vi "XW_Tutu_Chevray.vi"() -> (5 "Plug in titles":string[](array[string]), 7 "Plug in values":string[](array[string]))   [LabVIEW 2021]
uses:
  Controls/Inst_type.ctl
  Controls/In_Range.ctl
  Globals/Meas_global.vi
  <vilib>/Utility/file.llb/Read From Spreadsheet File (string).vi
panel:
  out "Calib Index":i32
  out "Third":dbl format="%#.3f"
  out "Filename":string
  out "Third Component":path
  out "U index":i32
  out "Log Row":i32
  out "2nd Comp":string
  out "1st Comp":string
  out "Iterations":i32
  out "Results table":string[][](table)
  out "Psi 2":dbl=-999.0 format="%.2f"
  out "Psi 1":dbl=-999.0 format="%.2f"
  out "UW":bool
  in  "constants":T1={"u'/U"=0.5, "v'/U"=0.4, "w'/U"=0.4, "rho"=0.5, "alpha1"=0.0, "alpha2"=0.0} {"alpha2" format="%.2f"; "alpha1" format="%.2f"; "rho" format="%.2f"; "w'/U" format="%.2f"; "v'/U" format="%.2f"; "u'/U" format="%.2f"}
  in  "u*, v* limits":T2={"u* low"=0.4, "u* high"=1.8, "v* low"=-0.6, "v* high"=0.8} {"v* high" format="%.2f"; "v* low" format="%.2f"; "u* high" format="%.2f"; "u* low" format="%.2f"}
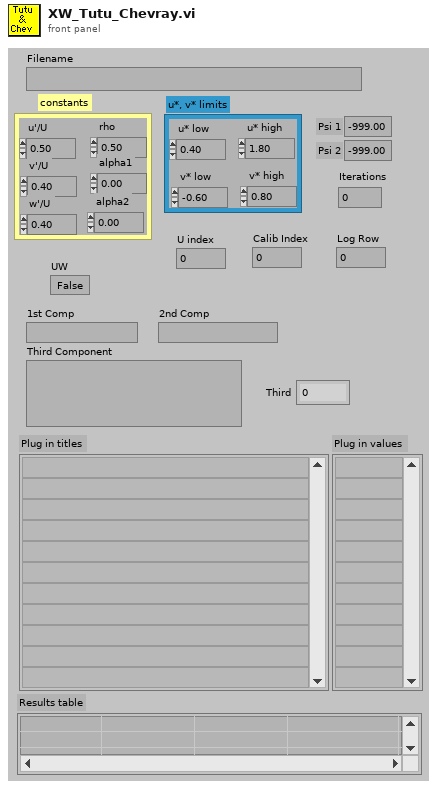
[diagram p1: front panel]
types:
  T1 = cluster{"u'/U":dbl, "v'/U":dbl, "w'/U":dbl, "rho":dbl, "alpha1":dbl, "alpha2":dbl}
  T2 = cluster{"u* low":dbl, "u* high":dbl, "v* low":dbl, "v* high":dbl}
  T3 = typedef "Analysis_info_cluster.ctl" = cluster{"Colour":u32, "Inst type":T4, "Inst name":string, "Symbol":string, "Code name":string, "Extra Info":string, "Inst Array":T5, "Extra Titles":string[], "Extra Values":string[], "U":dbl, "u^2":dbl, "u^3":dbl, "u^4":dbl, "Skew_u":dbl, "Kurt_u":dbl, "Sd Error in Mean":dbl, "% u'/U":dbl, "X":dbl, "Y":dbl, "Z":dbl, "Timescale integral Estimate":dbl, "Sd Error in Variance":dbl, "Calib File":path, "Calib Constants":dbl[], "Output Position":bool, "Stats":enum16{"None", "Basic", "Full"}, "Av Sampling Rate":dbl, "Av No of Samples":dbl, "Total Meas Time (s)":dbl, "ADAM Ch Name":string, "Max value":dbl, "Min value":dbl, "Req Sample Rate Hz":dbl, "Sync Delay Time (s)":dbl, "Ch No":i16, "Device":string, "Use Latest Calib":bool, "Port":string, "Metadata Ch Names":string[], "Metadata Ch Values":string[], "Label":string}
  T4 = typedef "Inst_type.ctl" = enum16{"Raw voltage", "Raw with zero offsetting", "Propeller anemometer", "Pressure Transducer", "Pitot-static tube", "Hot wire", "Cross wire 1", "Cross wire 2", "Generic Linear", "Generic Polynomial", "Generic BackPoly", "Fast FID", "Thermocouple", "Cold wire", "Pulsed Wire", "LDA Vel", "LDA Tran time", "LDA Arr time", "Microphone"}
  T5 = typedef "Instrument_Array.ctl" = enum16{"PWA", "LDA", "Analogue"}
  T6 = typedef "In_Range.ctl" = enum16{"%", "±", "% & ±"}
  T7 = enum16{"Save no data", "Save data in new files", "Save data in existing files"}
  T8 = typedef "Time_Trace_Cluster.ctl" = cluster{"Weighting":dbl[], "Voltage":dbl[], "Eng Values":dbl[]}
  T9 = typedef "Cross_Moments_Shift_Cluster.ctl" = cluster{"Stats":dbl[], "Resampled No of Samples":i32, "Resampled delta T":dbl, "Cross Correlation":dbl[]}
  T10 = typedef "Shift_Cluster.ctl" = cluster{"Stats":dbl[], "Spectra_Auto":dbl[], "Histogram":dbl[], "Hist Max":dbl, "Hist Min":dbl, "No of Samples":i32, "No in plume":i32, "Weight sum":dbl, "No Of Hist bins":i32, "TimeTrace Max":dbl, "Time Trace Min":dbl, "Trace St Deviation":dbl}
  T11 = typedef "Correlation_cluster1.ctl" = cluster{"U inst":string, "uw":dbl, "u^2w":dbl, "uw^2":dbl, "uw/u'w'":dbl, "W inst":string, "uw^3":dbl, "u^3w":dbl, "u^2w^2":dbl, "Index U":i32, "Index W":i32, "Error info":string[], "Paired Sampling Rate (Hz)":dbl, "u^2 Paired":dbl, "w^2 Paired":dbl, "Time Window (ms)":dbl}
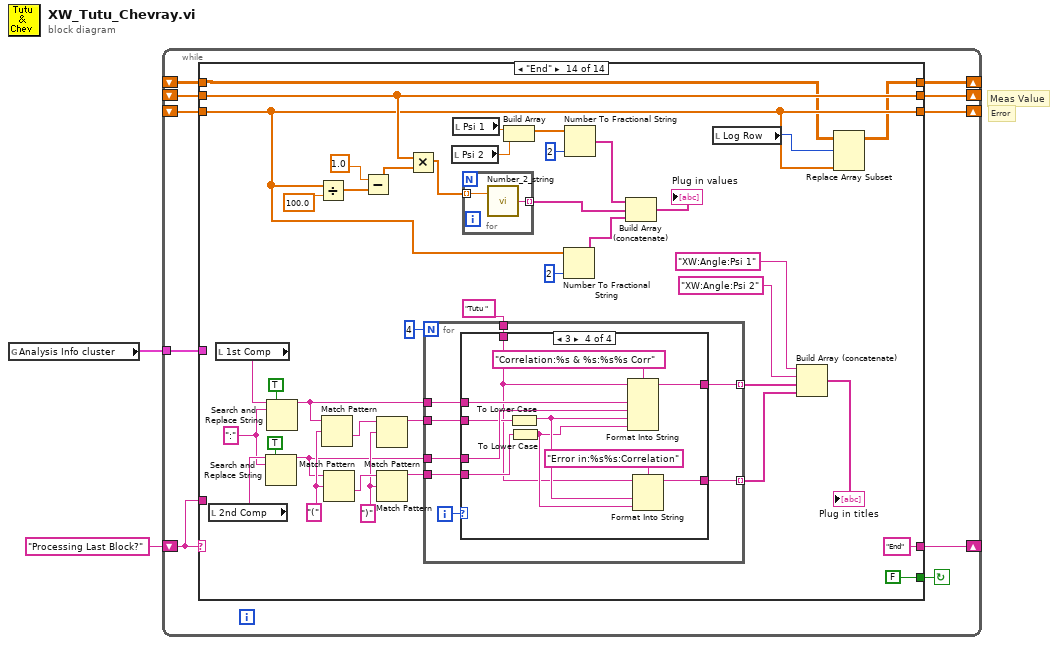
[diagram p0: block diagram]
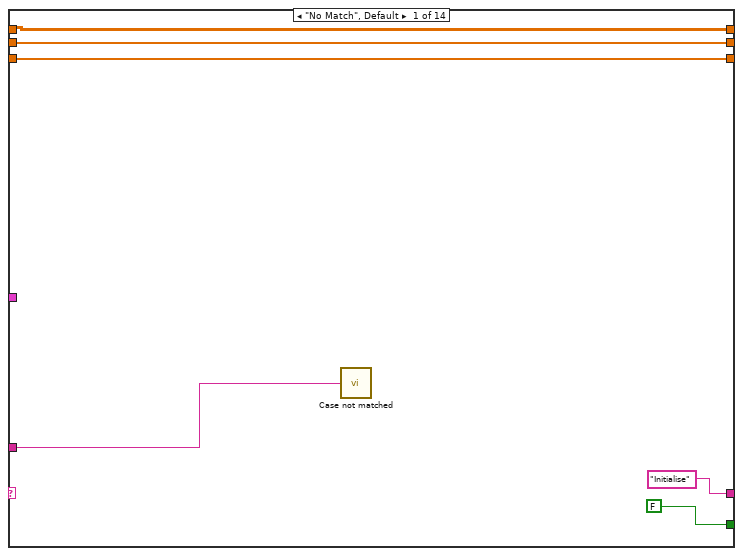
[diagram p2: hidden frame]
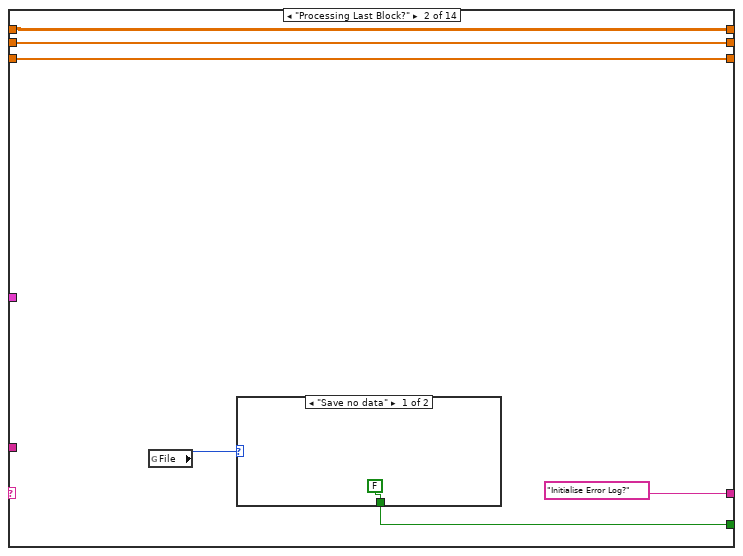
[diagram p3: hidden frame]
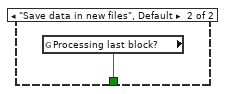
[diagram p4: hidden frame]
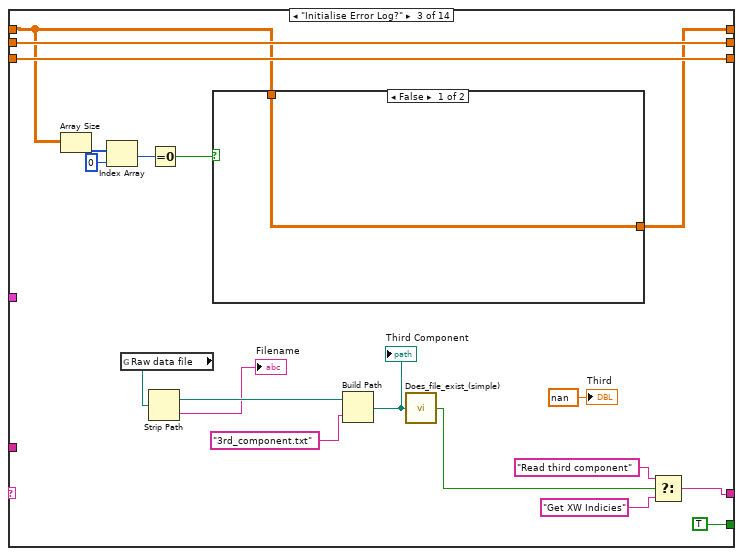
[diagram p5: hidden frame]
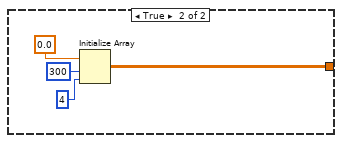
[diagram p6: hidden frame]
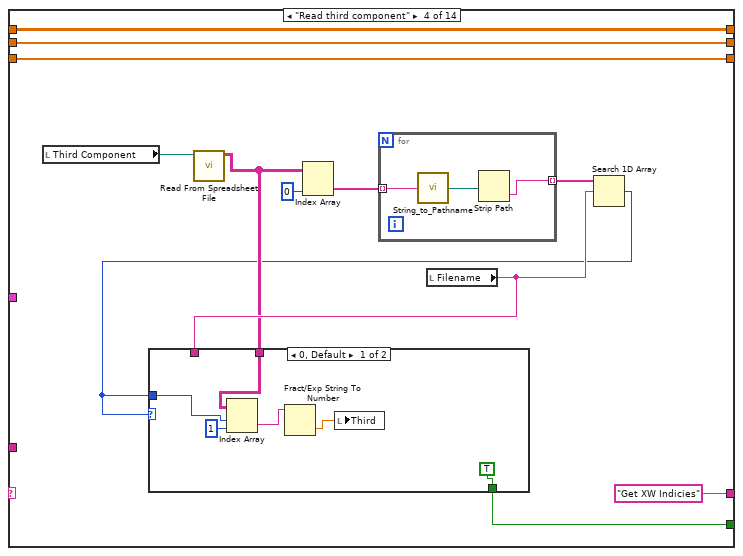
[diagram p7: hidden frame]
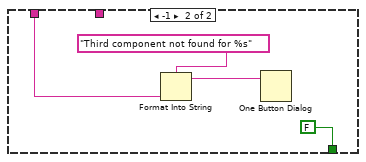
[diagram p8: hidden frame]
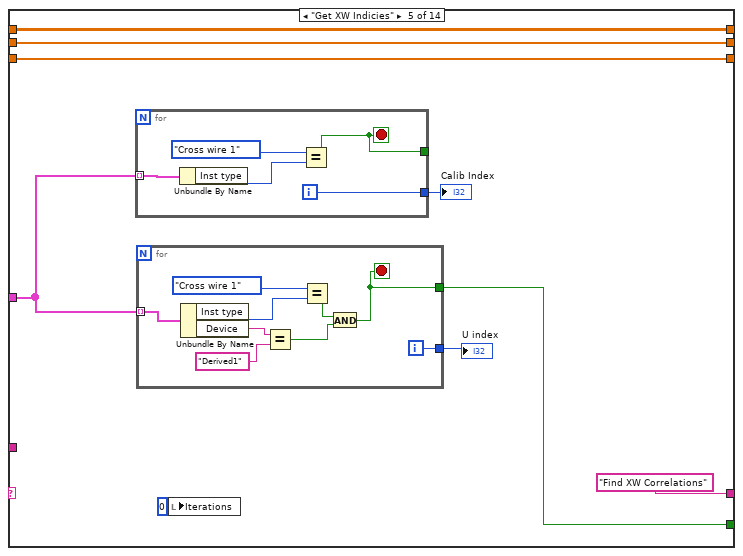
[diagram p9: hidden frame]
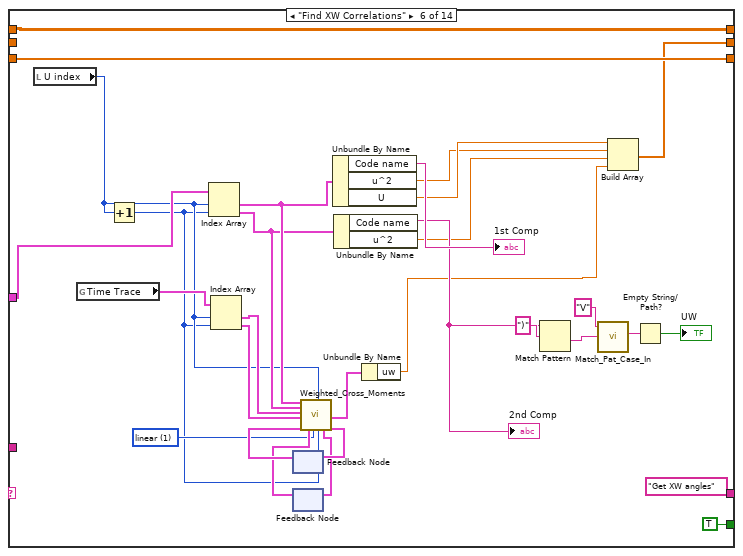
[diagram p10: hidden frame]
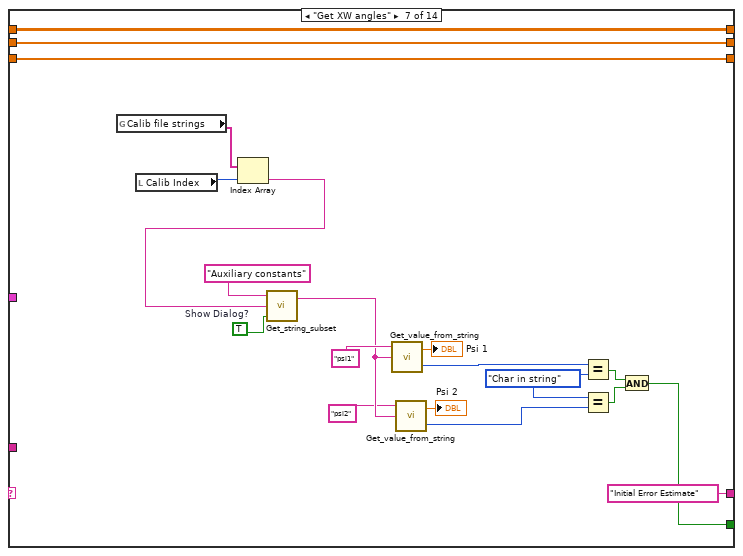
[diagram p11: hidden frame]
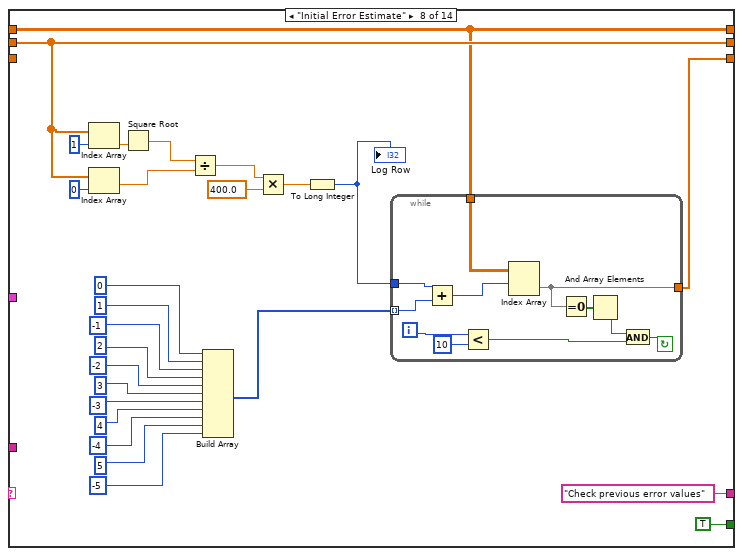
[diagram p12: hidden frame]
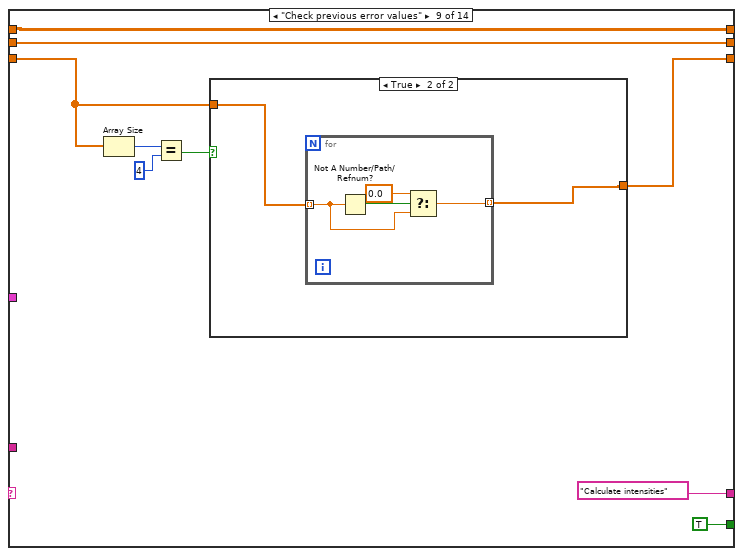
[diagram p13: hidden frame]
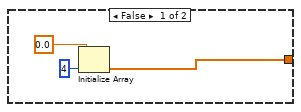
[diagram p14: hidden frame]
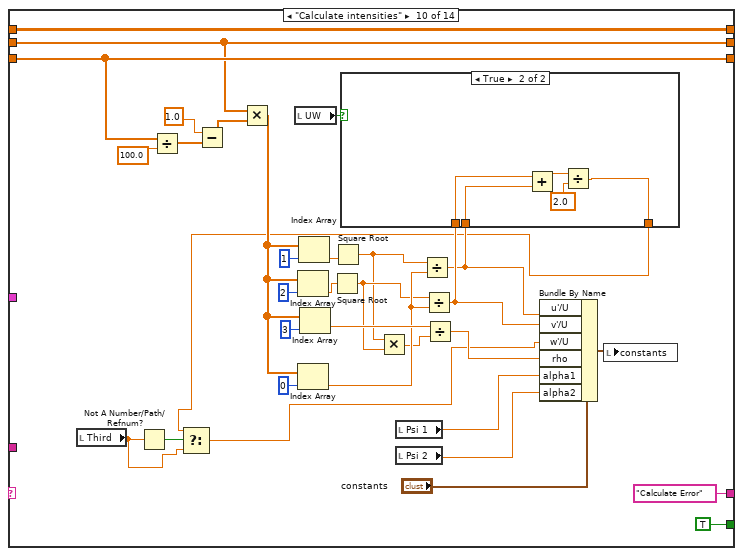
[diagram p15: hidden frame]
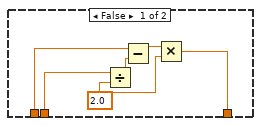
[diagram p16: hidden frame]
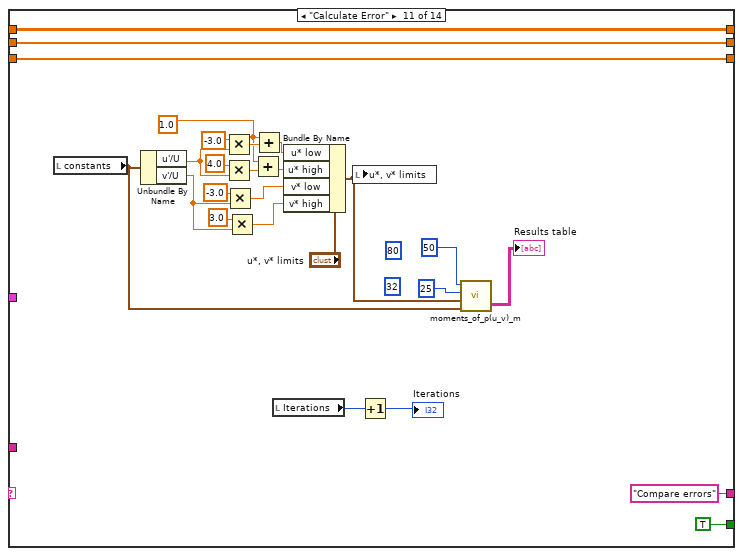
[diagram p17: hidden frame]
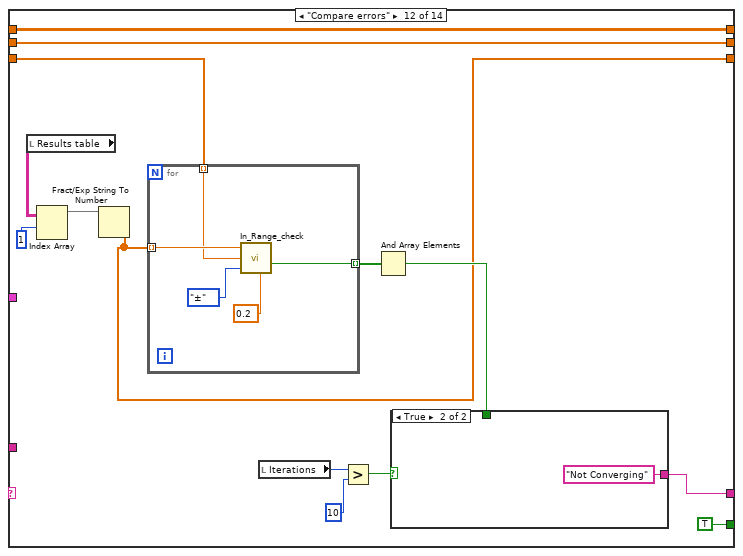
[diagram p18: hidden frame]
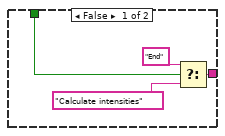
[diagram p19: hidden frame]
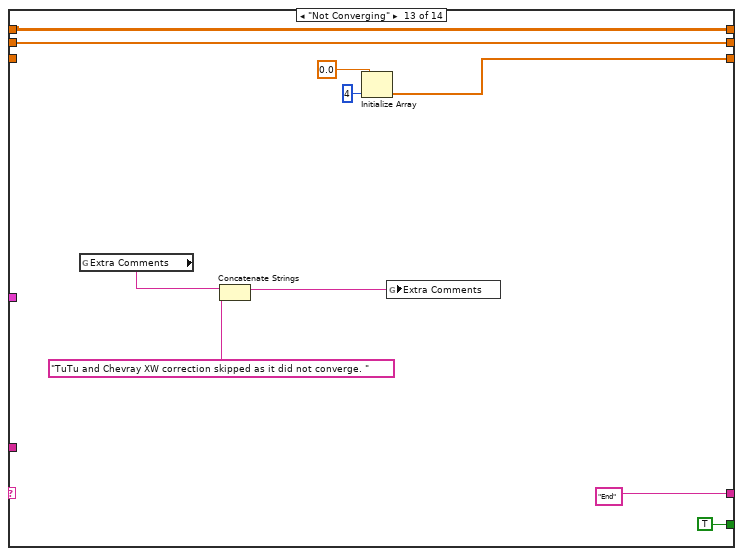
[diagram p20: hidden frame]
diagram:
  # "Error"
  # "Meas Value"
  n1 = global read "Meas_global.vi" "Analysis Info cluster"() -> (w1:T3[])
  n2 = while {
    tunnel: w1 -> [w6]
    shift-left: _ -> [w5]
    shift-right: [w7] -> _
    shift-left: _ -> [w8]
    shift-right: [w9] -> _
    shift-left: "Processing Last Block?" -> [w10]
    shift-right: [w11] -> _
    shift-right: [w3] -> _
    shift-left: _ -> [w4]
    stop <- w12 continue-if-true
    n3 = case shown="\"End\"" w10 {
      tunnel: [FALSE w23 TRUE ("Processing last block?") w53 w77 TRUE ("Processing last block?") w131 TRUE ("Processing last block?") TRUE ("Processing last block?") TRUE ("Processing last block?") TRUE ("Processing last block?") TRUE ("Processing last block?") TRUE ("Processing last block?") FALSE ("Processing last block?")] -> w12
      tunnel: ["Initialise" "Initialise Error Log?" w29 "Get XW Indicies" "Find XW Correlations" "Get XW angles" "Initial Error Estimate" "Check previous error values" ("f") "Calculate intensities" "Calculate Error" "Compare errors" w282 "End" "End"] -> w11
      tunnel: w10 -> [w13 _ _ _ _ _ _ _ _ _ _ _ _ _]
      tunnel: [w16 w22 w45 w61 w83 w119 w139 w167 w194 w228 w273 w287 w307 w342] -> w9
      tunnel: w8 -> [w16 w22 w45 w61 w83 _ w139 w167 w194 w228 w273 w287 w307 w342]
      tunnel: [w15 w20 w44 w60 w82 w127 w138 w161 w190 w233 w253 w278 w303 w321] -> w7
      tunnel: w6 -> [_ _ _ _ w79 w114 _ _ _ _ _ _ _ _]
      tunnel: w5 -> [w15 w20 w44 w60 w82 w127 w138 _ w189 w233 w253 w285 _ w321]
      tunnel: [w14 w19 w38 w62 w81 w115 w130 w163 w187 w208 w248 w274 w298 w320] -> w3
      tunnel: w4 -> [w14 w19 w37 w62 w81 w115 w130 w163 w187 w208 w248 w274 w298 w319]
      frame "No Match", Default {
        n4 = call "Case not matched.vi"("Case Name not Matched"=w13) -> ()
      }
      frame "Processing Last Block?" {
        n5 = global read "Meas_global.vi" "File"() -> (w21:T7)
        n6 = case shown="\"Save no data\"" w21 {
          tunnel: [FALSE ("Processing last block?") w26] -> w23
          frame "Save no data" {
          }
          frame "Save data in new files", Default {
            n7 = global read "Meas_global.vi" "Processing last block?"() -> (w26:bool)
          }
        }
      }
      frame "Initialise Error Log?" {
        n8 = Array Size(array=w37) -> (size(s)=w42:i32[])
        n9 = Index Array(array=w42, index=0) -> (element=w40:i32)
        n10 = global read "Meas_global.vi" "Raw data file"() -> (w36:path)
        n11 = Strip Path(path=w36) -> (stripped path=w35:path, name=→"Filename":string)
        n12 = Equal To 0?(x=w40) -> (x = 0?=w39:bool)
        n13 = case shown="False" w39 {
          tunnel: [w46 w47] -> w38
          tunnel: w37 -> [w46 _]
          frame False {
          }
          frame True {
            n14 = Initialize Array(0.0, 300 ("dimension size"), 4 ("dimension size")) -> (w47:dbl[][])
          }
        }
        n15 = Build Path(base path=w35, name or relative path="3rd_component.txt") -> (appended path=w33:path)
        "Third Component" <- w33
        n16 = call "Does_file_exist_(simple).vi"("Pathname"=w33) -> ("exists?"=w30:bool)
        n17 = Select(t="Read third component", s=w30, f="Get XW Indicies") -> (s? t:f=w29:string)
        "Third" <- nan ("Third")
      }
      frame "Read third component" {
        n18 = local read "Third Component"() -> (w58:path)
        n19 = call-poly <vilib>:"Read From Spreadsheet File.vi"("file path (dialog if empty)"=w58) -> ("all rows"=w52:string[][])  [unwired: 3 in, 7 out]
        n20 = Index Array(array=w52, index (col)=0 ("disabled index (col)")) -> (element=w56:string[])  [unwired: 1 in]
        n21 = for {
          tunnel: w56 -> [w75] mode=indexing
          tunnel: [w73] -> w55 mode=indexing
          n22 = call "String_to_Pathname.vi"("Input String"=w75) -> ("path"=w74:path)
          n23 = Strip Path(path=w74) -> (name=w73:string)  [unwired: 1 out]
        }
        n24 = local read "Filename"() -> (w54:string)
        n25 = Search 1D Array(1D array=w55, element=w54) -> (index of element=w51:i32)  [unwired: 1 out]
        n26 = case shown="0, Default" w51 {
          tunnel: w54 -> [_ w72]
          tunnel: [TRUE ("Processing last block?") FALSE ("Processing last block?")] -> w53
          tunnel: w52 -> [w66 _]
          tunnel: w51 -> [w65 _]
          frame 0, Default {
            n27 = Index Array(array=w66, index (row)=w65, index (col)=1 ("disabled index (col)")) -> (element=w64:string)
            n28 = Fract/Exp String To Number(string=w64) -> (number=w63:dbl)  [unwired: 4 out]
            n29 = local write "Third"(w63) -> ()
          }
          frame -1 {
            n30 = Format Into String(format string="Third component not found for %s" ("message"), w72) -> (resulting string=w70:string)  [unwired: 2 in, 1 out]
            n31 = One Button Dialog(message=w70) -> ()  [unwired: 2 out]
          }
        }
      }
      frame "Get XW Indicies" {
        n32 = for {
          tunnel: [w95] -> _
          tunnel: w79 -> [w97] mode=indexing
          tunnel: [w94] -> w76
          i -> [w94]
          stop <- w95 stop-if-true
          n33 = Unbundle By Name(w97) -> ("Inst type"=w98:T4)
          n34 = Equal?(x=Inst_type."Cross wire 1" ("Inst type"), y=w98) -> (x = y?=w95:bool)
        }
        "Calib Index" <- w76
        n35 = for {
          tunnel: [w86] -> w77
          tunnel: w79 -> [w92] mode=indexing
          tunnel: [w85] -> w78
          i -> [w85]
          stop <- w86 stop-if-true
          n36 = Unbundle By Name(w92) -> ("Inst type"=w93:T4, "Device"=w90:string)
          n37 = Equal?(x=w90, y="Derived1") -> (x = y?=w87:bool)
          n38 = Equal?(x=Inst_type."Cross wire 1" ("Inst type"), y=w93) -> (x = y?=w88:bool)
          n39 = And(x=w88, y=w87) -> (x .and. y?=w86:bool)
        }
        "U index" <- w78
        n40 = local write "Iterations"(0 ("Iterations")) -> ()
      }
      frame "Find XW Correlations" {
        w101 = 1 items=["nearest", "linear", "spline", "cubic Hermite", "Lagrange"] ("interp. method")
        n41 = local read "U index"() -> (w100:i32)
        n42 = global read "Meas_global.vi" "Time Trace"() -> (w113:T8[])
        n43 = Increment(x=w100) -> (x+1=w99:i32)
        n44 = Index Array(array=w114, index #1=w100, index #2=w99) -> (element #1=w112:T3, element #2=w111:T3)
        n45 = Index Array(array=w113, index #1=w100, index #2=w99) -> (element #1=w110:T8, element #2=w109:T8)
        n46 = feedback #1() -> (w107:T9)  [unwired: 1 in]
        n47 = feedback #2() -> (w106:T10)  [unwired: 1 in]
        n48 = call "Weighted_Cross_Moments.vi"("AI Cluster 1"=w112, "AI Cluster 2"=w111, "Time Cluster 1"=w110, "Time Cluster 2"=w109, "Shift Cluster In"=w107, "Shift Input"=w106, "interp. method"=w101, "Index1"=w100, "Index2"=w99) -> ("Shift Output"=w105:T10, "output cluster"=w104:T11, "Shift Cluster Out"=w108:T9)  [unwired: 8 in]
        n49 = feedback-in #1(w108) -> ()
        n50 = feedback-in #2(w105) -> ()
        n51 = Unbundle By Name(w112) -> ("Code name"=→"1st Comp":string, "u^2"=w116:dbl, "U"=w118:dbl)
        n52 = Unbundle By Name(w111) -> ("Code name"=w124:string, "u^2"=w117:dbl)
        "2nd Comp" <- w124
        n53 = Unbundle By Name(w104) -> ("uw"=w103:dbl)
        n54 = Match Pattern(string=w124, regular expression=")") -> (after substring=w122:string)  [unwired: 4 out]
        n55 = call "Match_Pat_Case_In.vi"("String to match"="V" ("regular expression"), "String"=w122) -> ("Matched string"=w121:string)  [unwired: 1 in, 3 out]
        n56 = Build Array(w118, w116, w117, w103) -> (w119:dbl[])
        n57 = Empty String/Path?(string/path=w121) -> (empty?=→"UW":bool)
      }
      frame "Get XW angles" {
        w136 = enum16{"Char in string", "Char not in string"}."Char in string" ("Status")
        w146 = TRUE  # Show Dialog?
        n58 = global read "Meas_global.vi" "Calib file strings"() -> (w148:string[])
        n59 = local read "Calib Index"() -> (w129:i32)
        n60 = Index Array(array=w148, index=w129) -> (element=w145:string)
        n61 = call "Get_string_subset.vi"("Show Dialog?"=w146, "String to split"=w145, "File Label"="Auxiliary constants") -> ("Output string"=w143:string)  [unwired: 1 in, 1 out]
        n62 = call "Get_value_from_string.vi"("Input string"=w143, "Variable name"="psi1") -> ("Status"=w135:enum16{"Char in string", "Char not in string"}, "Value"=→"Psi 1":dbl)  [unwired: 1 in]
        n63 = call "Get_value_from_string.vi"("Input string"=w143, "Variable name"="psi2") -> ("Status"=w134:enum16{"Char in string", "Char not in string"}, "Value"=→"Psi 2":dbl)  [unwired: 1 in]
        n64 = Equal?(x=w135, y=w136) -> (x = y?=w132:bool)
        n65 = Equal?(x=w136, y=w134) -> (x = y?=w133:bool)
        n66 = And(x=w132, y=w133) -> (x .and. y?=w131:bool)
      }
      frame "Initial Error Estimate" {
        n67 = Index Array(array=w167, index=1 ("Index")) -> (element=w169:dbl)
        n68 = Index Array(array=w167, index=0 ("Index")) -> (element=w165:dbl)
        n69 = Square Root(x=w169) -> (sqrt(x)=w166:dbl)
        n70 = Divide(x=w166, y=w165) -> (x/y=w164:dbl)
        n71 = Build Array(0, 1, -1, 2, -2, 3, -3, 4, -4, 5, -5) -> (w149:i32[])
        n72 = Multiply(x=w164, y=400.0) -> (x*y=w172:dbl)
        n73 = To Long Integer(number=w172) -> (32bit integer=w162:i32)
        "Log Row" <- w162
        n74 = while {
          tunnel: w163 -> [w185]
          tunnel: w162 -> [w184]
          tunnel: [w181] -> w161
          tunnel: w149 -> [w183] mode=indexing
          i -> [w177]
          stop <- w178 continue-if-true
          n75 = Add(x=w184, y=w183) -> (x+y=w182:i32)
          n76 = Less?(x=w177, y=10) -> (x < y?=w175:bool)
          n77 = Index Array(array=w185, index (row)=w182) -> (element=w181:dbl[])  [unwired: 1 in]
          n78 = Equal To 0?(x=w181) -> (x = 0?=w180:bool[])
          n79 = And Array Elements(Boolean array=w180) -> (logical AND=w179:bool)
          n80 = And(x=w179, y=w175) -> (x .and. y?=w178:bool)
        }
      }
      frame "Check previous error values" {
        n81 = Array Size(array=w189) -> (size(s)=w193:i32)
        n82 = Equal?(x=w193, y=4) -> (x = y?=w191:bool)
        n83 = case shown="True" w191 {
          tunnel: [w195 w198] -> w190
          tunnel: w189 -> [_ w199]
          frame False {
            n84 = Initialize Array(0.0, 4 ("Dimension Size")) -> (w195:dbl[])
          }
          frame True {
            n85 = for {
              tunnel: w199 -> [w201] mode=indexing
              tunnel: [w200] -> w198 mode=indexing
              n86 = Not A Number/Path/Refnum?(number/path/refnum=w201) -> (NaN/Path/Refnum?=w203:bool)
              n87 = Select(t=0.0, s=w203, f=w201) -> (s? t:f=w200:dbl)
            }
          }
        }
      }
      frame "Calculate intensities" {
        n88 = local read "Third"() -> (w204:dbl)
        n89 = Not A Number/Path/Refnum?(number/path/refnum=w204) -> (NaN/Path/Refnum?=w207:bool)
        n90 = Divide(x=w233, y=100.0) -> (x/y=w231:dbl[])
        n91 = Subtract(x=1.0, y=w231) -> (x-y=w229:dbl[])
        n92 = Multiply(x=w228, y=w229) -> (x*y=w222:dbl[])
        n93 = local read "UW"() -> (w213:bool)
        n94 = Index Array(array=w222, index=2 ("Index")) -> (element=w220:dbl)
        n95 = Index Array(array=w222, index=0 ("Index")) -> (element=w217:dbl)
        n96 = Index Array(array=w222, index=1 ("Index")) -> (element=w221:dbl)
        n97 = Index Array(array=w222, index=3 ("Index")) -> (element=w218:dbl)
        n98 = Square Root(x=w220) -> (sqrt(x)=w216:dbl)
        n99 = Square Root(x=w221) -> (sqrt(x)=w215:dbl)
        n100 = Multiply(x=w215, y=w216) -> (x*y=w214:dbl)
        n101 = local read "Psi 1"() -> (w234:dbl)
        n102 = local read "Psi 2"() -> (w235:dbl)
        n103 = Divide(x=w215, y=w217) -> (x/y=w211:dbl)
        n104 = Divide(x=w216, y=w217) -> (x/y=w212:dbl)
        n105 = case shown="True" w213 {
          tunnel: w212 -> [w238 w244]
          tunnel: w211 -> [w237 w243]
          tunnel: [w239 w245] -> w206
          frame False {
            w240 = 2.0 ("y")
            n106 = Divide(x=w237, y=w240) -> (x/y=w242:dbl)
            n107 = Subtract(x=w238, y=w242) -> (x-y=w241:dbl)
            n108 = Multiply(x=w241, y=w240) -> (x*y=w239:dbl)
          }
          frame True {
            n109 = Add(x=w244, y=w243) -> (x+y=w247:dbl)
            n110 = Divide(x=w247, y=2.0) -> (x/y=w245:dbl)
          }
        }
        n111 = Select(t=w206, s=w207, f=w204) -> (s? t:f=w205:dbl)
        n112 = Divide(x=w218, y=w214) -> (x/y=w219:dbl)
        n113 = Bundle By Name(cluster="constants", "u'/U"=w211, "v'/U"=w212, "w'/U"=w205, "rho"=w219, "alpha1"=w234, "alpha2"=w235) -> (w227:T1)
        n114 = local write "constants"(w227) -> ()
      }
      frame "Calculate Error" {
        (unwired) i16 32 ("grid size for z*")
        (unwired) i16 80 ("grid size for u* and v*")
        w260 = 1.0
        n115 = local read "constants"() -> (w256:T1)
        n116 = Unbundle By Name(w256) -> ("u'/U"=w262:dbl, "v'/U"=w261:dbl)
        n117 = Multiply(x=-3.0, y=w262) -> (x*y=w268:dbl)
        n118 = Multiply(x=4.0, y=w262) -> (x*y=w267:dbl)
        n119 = Multiply(x=-3.0, y=w261) -> (x*y=w264:dbl)
        n120 = Multiply(x=3.0, y=w261) -> (x*y=w263:dbl)
        n121 = Add(x=w260, y=w267) -> (x+y=w265:dbl)
        n122 = Add(x=w260, y=w268) -> (x+y=w266:dbl)
        n123 = local read "Iterations"() -> (w250:i32)
        n124 = Bundle By Name(cluster="u*, v* limits", "u* low"=w266, "u* high"=w265, "v* low"=w264, "v* high"=w263) -> (w255:T2)
        n125 = local write "u*, v* limits"(w255) -> ()
        n126 = Increment(x=w250) -> (x+1=→"Iterations":i32)
        n127 = call "moments_of_p(u_v)_m.vi"("constants"=w256, "u*, v* limits"=w255, "grid size for z*"=i16 25, "grid size for u* and v*"=i16 50) -> ("Results table"=→"Results table":string[][])  [unwired: 7 out]
      }
      frame "Compare errors" {
        n128 = local read "Results table"() -> (w279:string[][])
        n129 = Index Array(array=w279, index (row)=1) -> (element=w280:string[])  [unwired: 1 in]
        n130 = Fract/Exp String To Number(string=w280) -> (number=w278:dbl[])  [unwired: 4 out]
        n131 = for {
          tunnel: w278 -> [w296] mode=indexing
          tunnel: w285 -> [w295] mode=indexing
          tunnel: [w293] -> w286 mode=indexing
          n132 = call "In_Range_check.vi"("±"=0.2, "Mode"=In_Range."±", "Value"=w295, "Setpoint"=w296) -> ("In Range"=w293:bool)  [unwired: 1 in, 2 out]
        }
        n133 = local read "Iterations"() -> (w277:i32)
        n134 = Greater?(x=w277, y=10) -> (0:w275:bool)
        n135 = And Array Elements(Boolean array=w286) -> (logical AND=w284:bool)
        n136 = case shown="True" w275 {
          tunnel: w284 -> [w291 _]
          tunnel: [w289 "Not Converging" ("f")] -> w282
          frame False {
            n137 = Select(t="End", s=w291, f="Calculate intensities") -> (s? t:f=w289:string)
          }
          frame True {
          }
        }
      }
      frame "Not Converging" {
        n138 = global read "Meas_global.vi" "Extra Comments"() -> (w301:string)
        n139 = Concatenate Strings(w301, "TuTu and Chevray XW correction skipped as it did not converge. " ("Format String")) -> (w299:string)
        n140 = Initialize Array(0.0, 4 ("Dimension Size")) -> (w303:dbl[])
        n141 = global write "Meas_global.vi" "Extra Comments"(w299) -> ()
      }
      frame "End" {
        w308 = ":" ("search string")
        w315 = "(" ("regular expression")
        w316 = ")" ("regular expression")
        n142 = local read "2nd Comp"() -> (w310:string)
        n143 = local read "1st Comp"() -> (w313:string)
        n144 = Search and Replace String(replace all?=TRUE ("replace all? (F)"), input string=w310, search string=w308) -> (result string=w309:string)  [unwired: 5 in, 3 out]
        n145 = Search and Replace String(replace all?=TRUE ("replace all? (F)"), input string=w313, search string=w308) -> (result string=w312:string)  [unwired: 5 in, 3 out]
        n146 = Divide(x=w321, y=100.0) -> (x/y=w345:dbl[])
        n147 = Match Pattern(string=w312, regular expression=w315) -> (after substring=w340:string)  [unwired: 4 out]
        n148 = Match Pattern(string=w309, regular expression=w315) -> (after substring=w339:string)  [unwired: 4 out]
        n149 = Subtract(x=1.0, y=w345) -> (x-y=w343:dbl[])
        n150 = Match Pattern(string=w340, regular expression=w316) -> (before substring=w338:string)  [unwired: 4 out]
        n151 = Match Pattern(string=w339, regular expression=w316) -> (before substring=w334:string)  [unwired: 4 out]
        n152 = Multiply(x=w342, y=w343) -> (x*y=w318:dbl[])
        n153 = for {
          N: 4 -> [_]
          tunnel: "Tutu " -> [w357]
          tunnel: w312 -> [w356]
          tunnel: w338 -> [w355]
          tunnel: [w354] -> w337 mode=indexing
          tunnel: [w353] -> w336 mode=indexing
          tunnel: w309 -> [w352]
          tunnel: w334 -> [w351]
          i -> [w358]
          n154 = case shown="3" w358 {
            tunnel: w357 -> [w359 w367 w375 w383]
            tunnel: w356 -> [w362 w372 _ w388]
            tunnel: w355 -> [w365 w369 _ w386]
            tunnel: [w361 w371 w380 w391] -> w354
            tunnel: [w360 w370 w379 w390] -> w353
            tunnel: w352 -> [_ _ w377 w387]
            tunnel: w351 -> [_ _ w376 w389]
            frame 0, Default {
              n155 = To Upper Case(1:w365) -> (0:w366:string)
              n156 = Format Into String(format string="Mean:%s:%s Corr" ("Format String"), initial string=w359, w362, w366) -> (resulting string=w360:string)  [unwired: 1 in, 1 out]
              n157 = Format Into String(format string="Error in:%s:Mean" ("Format String"), initial string=w359, w362) -> (resulting string=w361:string)  [unwired: 1 in, 1 out]
            }
            frame 1 {
              n158 = To Lower Case(string=w369) -> (all lower case string=w368:string)
              n159 = Format Into String(format string="Variance:%s:%s^2 Corr" ("Format String"), initial string=w367, w372, w368) -> (resulting string=w370:string)  [unwired: 1 in, 1 out]
              n160 = Format Into String(format string="Error in:%s:Variance" ("Format String"), initial string=w367, w372) -> (resulting string=w371:string)  [unwired: 1 in, 1 out]
            }
            frame 2 {
              n161 = To Lower Case(string=w376) -> (all lower case string=w378:string)
              n162 = Format Into String(format string="Variance:%s:%s^2 Corr" ("Format String"), initial string=w375, w377, w378) -> (resulting string=w379:string)  [unwired: 1 in, 1 out]
              n163 = Format Into String(format string="Error in:%s:Variance" ("Format String"), initial string=w375, w377) -> (resulting string=w380:string)  [unwired: 1 in, 1 out]
            }
            frame 3 {
              n164 = To Lower Case(string=w386) -> (all lower case string=w385:string)
              n165 = To Lower Case(string=w389) -> (all lower case string=w384:string)
              n166 = Format Into String(format string="Correlation:%s & %s:%s%s Corr" ("Format String"), initial string=w383, w388, w387, w385, w384) -> (resulting string=w390:string)  [unwired: 1 in, 1 out]
              n167 = Format Into String(format string="Error in:%s%s:Correlation" ("Format String"), initial string=w383, w385, w384) -> (resulting string=w391:string)  [unwired: 1 in, 1 out]
            }
          }
        }
        n168 = local read "Psi 2"() -> (w325:dbl)
        n169 = local read "Psi 1"() -> (w326:dbl)
        n170 = for {
          tunnel: w318 -> [w350] mode=indexing
          tunnel: [w349] -> w317 mode=indexing
          n171 = call "Number_2_string.vi"("number"=w350) -> ("String"=w349:string)  [unwired: 1 in]
        }
        n172 = Build Array(w326, w325) -> (w324:dbl[])
        n173 = Number To Fractional String(number=w321, precision (6)=i16 2) -> (F-format string=w331:string[])  [unwired: 2 out]
        n174 = Number To Fractional String(number=w324, precision (6)=i16 2) -> (F-format string=w323:string[])  [unwired: 2 out]
        n175 = Build Array (concatenate)(w323, w317, w331) -> (→"Plug in values":string[])
        n176 = local read "Log Row"() -> (w322:i32)
        n177 = Build Array (concatenate)("XW:Angle:Psi 1", "XW:Angle:Psi 2", w336, w337) -> (→"Plug in titles":string[])
        n178 = Replace Array Subset(array=w319, new element=w321, index (row)=w322) -> (w320:dbl[][])  [unwired: 1 in]
      }
    }
  }
